vi "Init AMG8833.vi"(8 "error in (no error)":errorcluster, 11 "AMG8833 8x8 Camera in":refnum<class "AMG8833 8x8 Camera.lvclass">) -> (0 "error out":errorcluster, 3 "AMG8833 8x8 Camera out":refnum<class "AMG8833 8x8 Camera.lvclass">)   [LabVIEW 2020, in "CTI-Peripheral.lvlib" / "AMG8833 8x8 Camera.lvclass"]
uses:
  AMG8833 8x8 Camera.lvclass
  AMG8833 8x8 Camera.lvclass/AMG8833 8x8 Camera.ctl
  CTI/I2C Connection/I2C Connection.lvclass/I2C Connection.ctl
  CTI/Session/I2C Write Data.vi
  CTI/Session/I2C Read Data.vi
  CTI/I2C Connection/I2C Connection.lvclass
panel:
  out "Thermistor Value":dbl
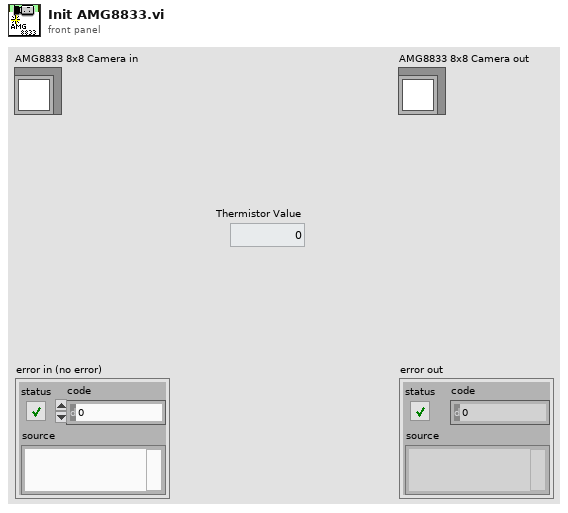
[diagram p1: front panel]
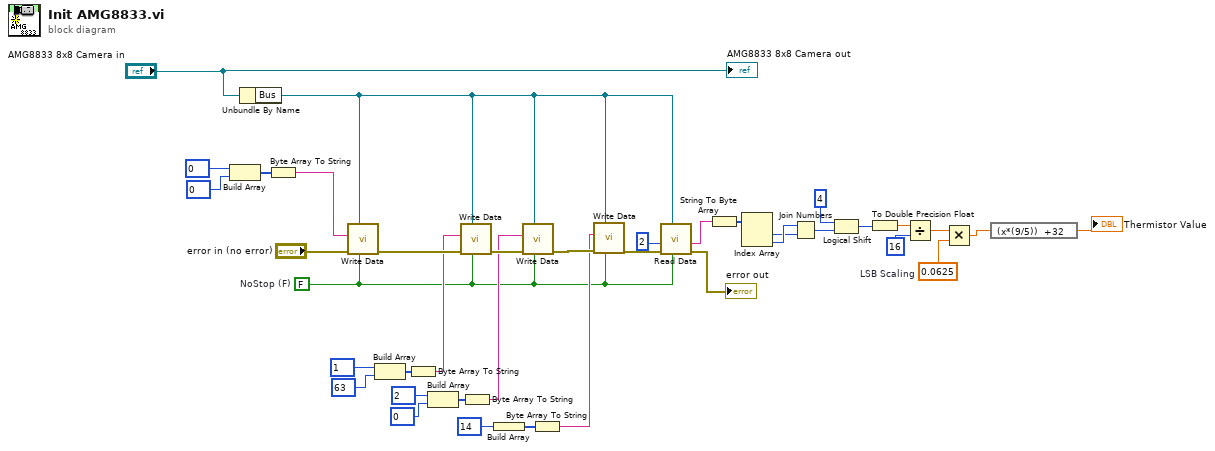
[diagram p0: block diagram]
diagram:
  w15 = 0.0625  # LSB Scaling
  w2 = FALSE  # NoStop (F)
  n1 = Build Array(u8 0 ("Address"), u8 0 ("Address")) -> (w35:u8[])
  n2 = Unbundle By Name("AMG8833 8x8 Camera in") -> ("Bus"=w3:refnum<class "I2C Connection.lvclass">)
  n3 = Byte Array To String(unsigned byte array=w35) -> (string=w14:string)
  n4 = call "Write Data.vi"("NoStop (F)"=w2, "I2C Connection"=w3, "error in (no error)"="error in (no error)", "Data"=w14) -> ("error out"=w13:errorcluster)  [unwired: 7 in]
  n5 = Build Array(u8 1 ("Address"), u8 63 ("Address")) -> (w34:u8[])
  n6 = Byte Array To String(unsigned byte array=w34) -> (string=w12:string)
  n7 = Build Array(u8 2 ("Address"), u8 0 ("Address")) -> (w29:u8[])
  n8 = call "Write Data.vi"("NoStop (F)"=w2, "I2C Connection"=w3, "error in (no error)"=w13, "Data"=w12) -> ("error out"=w11:errorcluster)  [unwired: 7 in]
  n9 = Byte Array To String(unsigned byte array=w29) -> (string=w10:string)
  n10 = Build Array(u8 14 ("Address")) -> (w27:u8[])
  n11 = call "Write Data.vi"("NoStop (F)"=w2, "I2C Connection"=w3, "error in (no error)"=w11, "Data"=w10) -> ("error out"=w9:errorcluster)  [unwired: 7 in]
  n12 = Byte Array To String(unsigned byte array=w27) -> (string=w8:string)
  n13 = call "Write Data.vi"("NoStop (F)"=w2, "I2C Connection"=w3, "error in (no error)"=w9, "Data"=w8) -> ("error out"=w6:errorcluster)  [unwired: 7 in]
  n14 = call "Read Data.vi"("NoStop (F)"=w2, "I2C Connection"=w3, "error in (no error)"=w6, "Len"=u8 2 ("Read Len")) -> ("error out"=→"error out":errorcluster, "Data"=w5:string)  [unwired: 6 in]
  n15 = String To Byte Array(string=w5) -> (unsigned byte array=w26:u8[])
  n16 = Index Array(array=w26) -> (element #1=w24:u8, element #2=w25:u8)  [unwired: 2 in]
  n17 = Join Numbers(hi=w25, lo=w24) -> ((hi.lo)=w17:u16)
  n18 = Logical Shift(y=i16 4, x=w17) -> (x << y=w20:u16)
  n19 = To Double Precision Float(number=w20) -> (double precision float=w21:dbl)
  n20 = Divide(x=w21, y=i16 16) -> (x/y=w23:dbl)
  n21 = Multiply(x=w23, y=w15) -> (x*y=w16:dbl)
  n22 = expression code="(x*(9/5))  +32"(w16) -> (→"Thermistor Value":dbl)
  "AMG8833 8x8 Camera out" <- "AMG8833 8x8 Camera in"
